vi "Tektronix_AWG Parse Binary AWG File.vi"() -> ()   [LabVIEW 2010]
doc: "Reads an array of data from a byte stream binary file. By default, the VI is configured to read 8-byte (data type DBL) Little Endian Data. To modify the way sample data is read from the file, change the Byte Order and the value of the Byte Size (normal sizes are 1, 2, 4, or 8). If you change the byte size, also change the representation of the Data Type constant (default is DBL) to coincide with the byte size (1 = I8, 2 = I16, 4 = I32, 8 = DBL). Use the Write Binary File VI in this LLB to create the file.\n\nThis example was built using LabVIEW 8.0"
panel:
  in  "Include Data Bytes as 2nd Column":bool
  out "error out":errorcluster
  in  "read file path (.awg)":path=path "c:/data/sequences/Setup1.awg"
  in  "Save As Text File?\n(will prompt for path)":bool
  out "Data":string[](array[string])
  out "Size in bytes":u32[](array[numeric])
  out "Name":string[](array[string])
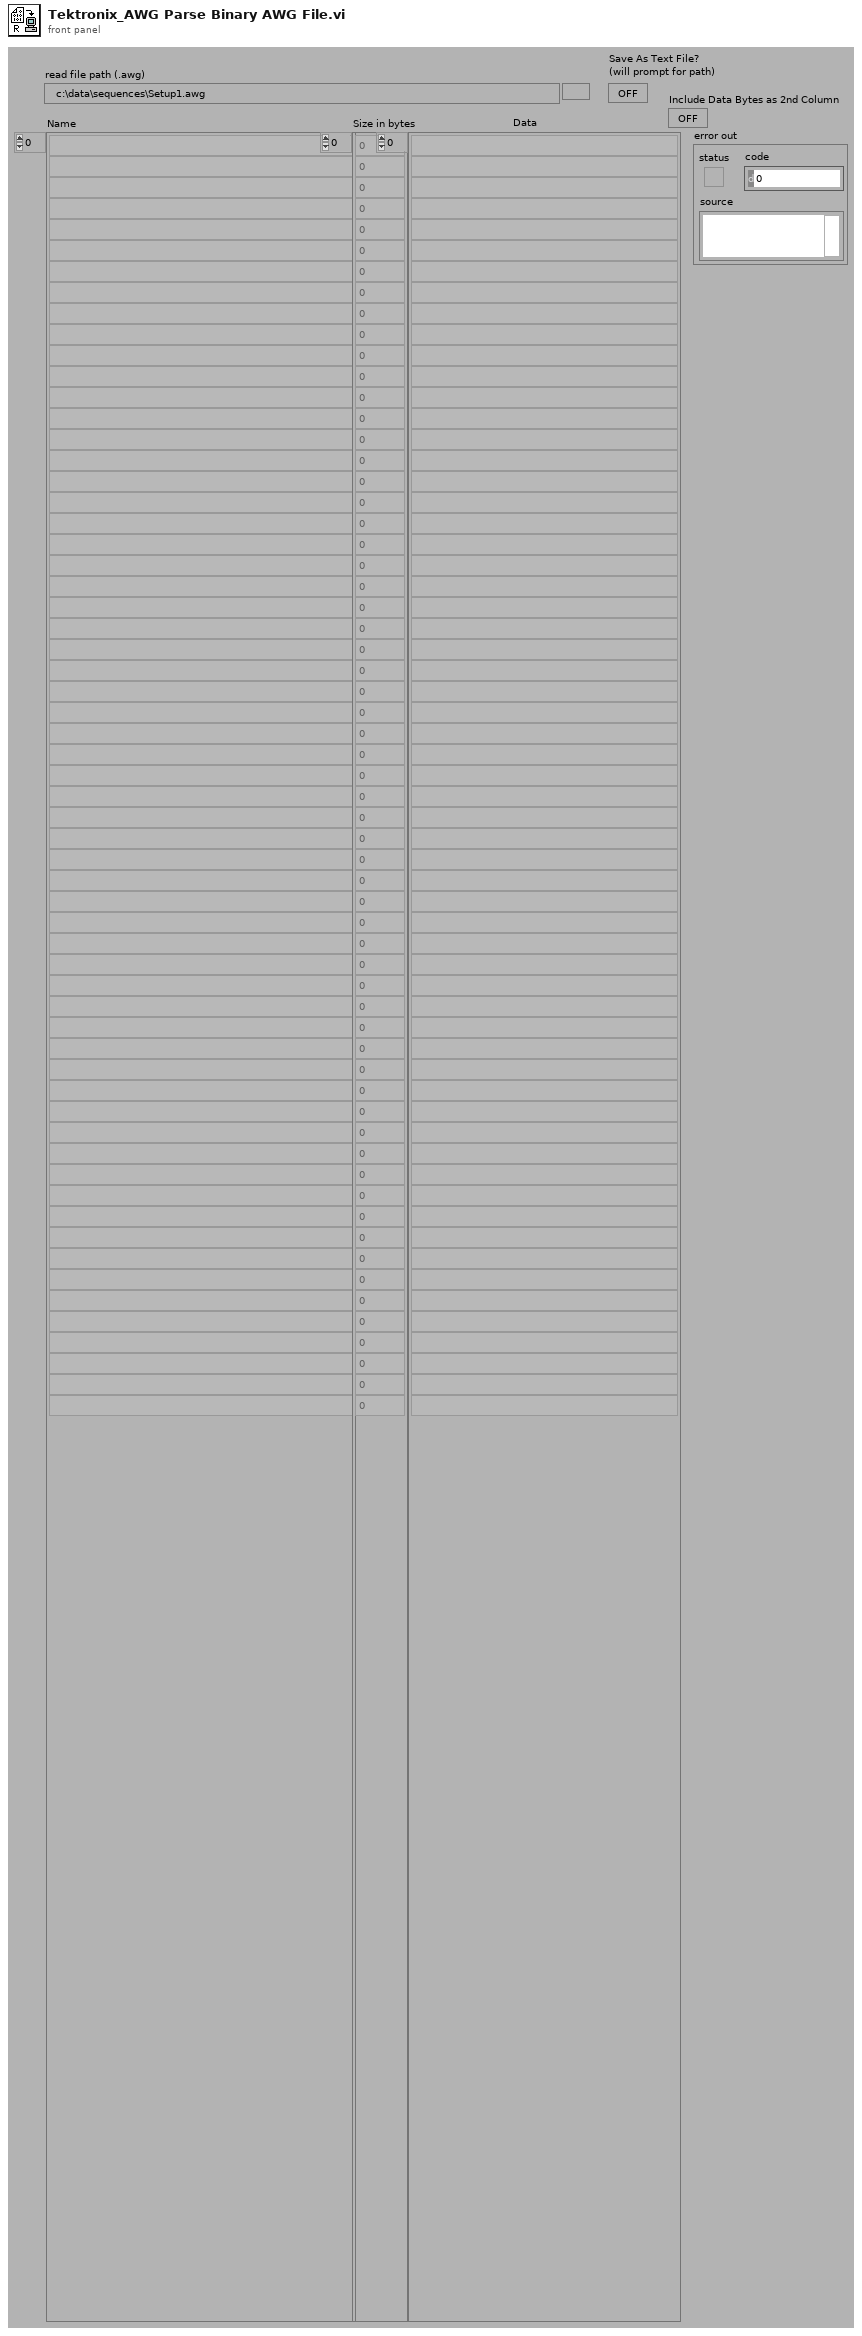
[diagram p1: front panel]
types:
  T1 = enum16{"open", "replace", "create", "open or create", "replace or create", "replace or create with confirmation"}
  T2 = enum16{"deny read/write", "deny write-only", "deny none"}
  T3 = enum16{"big-endian, network order", "native, host order", "little-endian"}
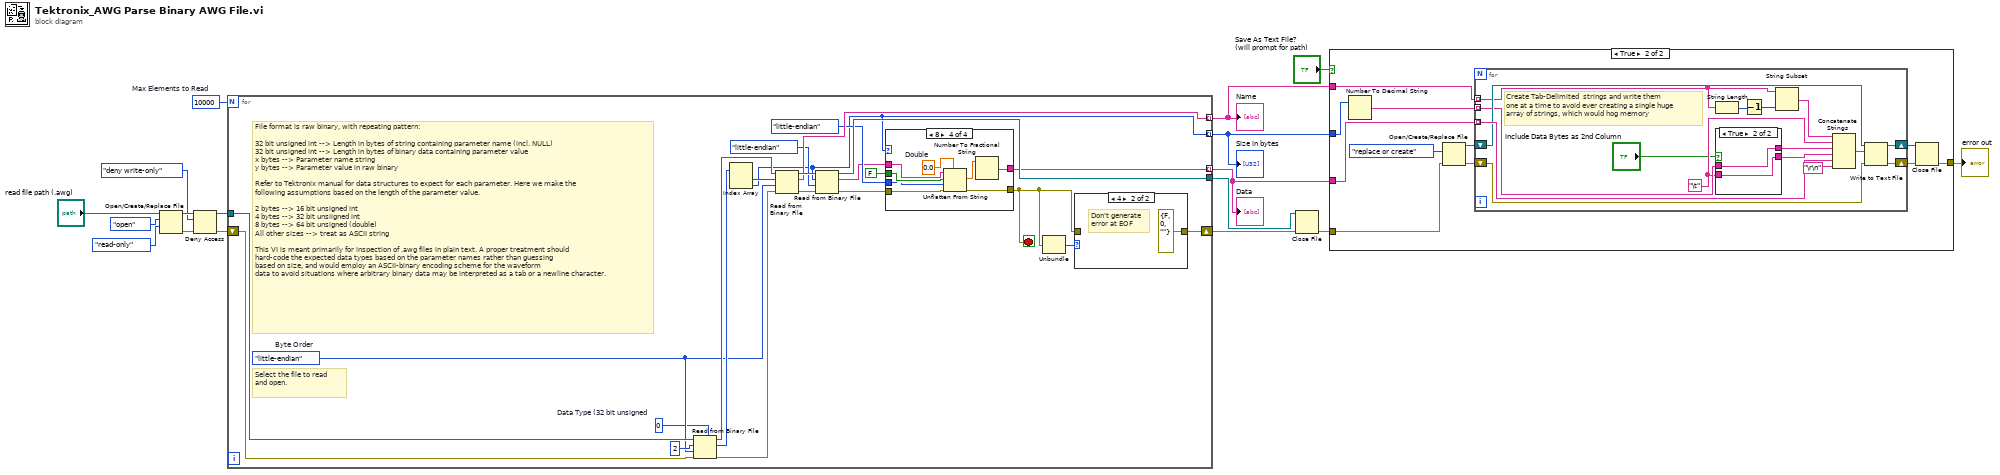
[diagram p0: block diagram]
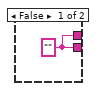
[diagram p3: hidden frame]
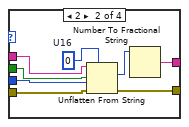
[diagram p6: hidden frame]
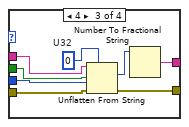
[diagram p7: hidden frame]
diagram:
  w7 = 10000  # Max Elements to Read
  n1 = Open/Create/Replace File(file path (use dialog)="read file path (.awg)", operation (0:open)=T1."open", access (0:read/write)=enum16{"read/write", "read-only", "write-only"}."read-only") -> (refnum out=w15:refnum<file>, error out=w16:errorcluster)  [unwired: 3 in, 1 out]
  n2 = Deny Access(4:w16, 6:T2."deny write-only" ("deny mode (0:deny read/write)"), 7:w15) -> (0:w11:errorcluster, 3:w12:refnum<file>)
  n3 = for {
    N: w7 -> [_]
    tunnel: w12 -> [w40]
    tunnel: [w32] -> w9
    tunnel: [w29] -> w6 mode=indexing
    tunnel: [w22] -> w5 mode=indexing
    tunnel: [w21] -> w4 mode=indexing
    shift-right: [w18] -> w8
    shift-left: w11 -> [w38]
    stop <- w19 stop-if-true
    w30 = T3."little-endian"  # Byte Order
    w28 = u32 0  # Data Type (32 bit unsigned
    # "File format is raw binary, with repeating pattern:\n\n32 bit unsigned int --> Length in bytes of string containing parameter name (incl. NULL)\n32 bit unsigned int --> Length in bytes of binary data containing parameter value\nx bytes --> Parameter name string\ny bytes --> Parameter value in raw binary\n\nRefer to Tektronix manual for data structures to expect for each parameter. Here we make the \nfollowing assumptions based on the length of the parameter value. \n\n2 bytes --> 16 bit unsigned int\n4 bytes --> 32 bit unsiigned int\n8 bytes --> 64 bit unsigned (double)\nAll other sizes --> treat as ASCII string\n\nThis VI is meant primarily for inspection of .awg files in plain text. A proper treatment should \nhard-code the expected data types based on the parameter names rather than guessing \nbased on size, and would employ an ASCII-binary encoding scheme for the waveform\ndata to avoid situations where arbitrary binary data may be interpreted as a tab or a newline character."
    # "Select the file to read and open."
    n4 = Read from Binary File(5:w28, 8:w38, 9:w30, 10:2 ("count (1)"), 11:w40) -> (0:w36:errorcluster, 2:w35:u32[], 3:w37:refnum<file>)  [unwired: 1 in, 1 out]
    n5 = Index Array(array=w35) -> (element #1=w31:u32, element #2=w22:u32)  [unwired: 2 in]
    n6 = Read from Binary File(8:w36, 9:w30, 10:w31, 11:w37) -> (0:w34:errorcluster, 2:w29:string, 3:w33:refnum<file>)  [unwired: 2 in, 1 out]
    n7 = Read from Binary File(8:w34, 9:T3."little-endian" ("byte order (0:big-endian, network order)"), 10:w22, 11:w33) -> (0:w23:errorcluster, 2:w24:string, 3:w32:refnum<file>)  [unwired: 2 in, 1 out]
    n8 = case shown="8" w22 {
      tunnel: FALSE ("data includes array or string size? (T)") -> [_ w52 w60 w68]
      tunnel: T3."little-endian" ("byte order (0:big-endian, network order)") -> [_ w51 w59 w67]
      tunnel: w24 -> [w43 w50 w58 w66]
      tunnel: w23 -> [w44 w49 w57 w65]
      tunnel: [w44 w48 w56 w64] -> w19
      tunnel: [w43 w45 w53 w61] -> w21
      frame 0, Default {
      }
      frame 2 {
        w47 = u16 0  # U16
        n9 = Unflatten From String(type=w47, binary string=w50, data includes array or string size? (T)=w52, byte order (0:big-endian, network order)=w51, error in (no error)=w49) -> (value=w46:u16, error out=w48:errorcluster)  [unwired: 1 out]
        n10 = Number To Fractional String(number=w46) -> (F-format string=w45:string)  [unwired: 3 in]
      }
      frame 4 {
        w55 = u32 0  # U32
        n11 = Unflatten From String(type=w55, binary string=w58, data includes array or string size? (T)=w60, byte order (0:big-endian, network order)=w59, error in (no error)=w57) -> (value=w54:u32, error out=w56:errorcluster)  [unwired: 1 out]
        n12 = Number To Fractional String(number=w54) -> (F-format string=w53:string)  [unwired: 3 in]
      }
      frame 8 {
        w63 = 0.0  # Double
        n13 = Unflatten From String(type=w63, binary string=w66, data includes array or string size? (T)=w68, byte order (0:big-endian, network order)=w67, error in (no error)=w65) -> (value=w62:dbl, error out=w64:errorcluster)  [unwired: 1 out]
        n14 = Number To Fractional String(number=w62) -> (F-format string=w61:string)  [unwired: 3 in]
      }
    }
    n15 = Unbundle(w19) -> ("code"=w20:i32)  [unwired: 2 out]
    n16 = case shown="4" w20 {
      tunnel: w19 -> [w41 _]
      tunnel: [w41 errorcluster {"status"=FALSE, "code"=0, "source"=""} ("error out")] -> w18
      frame 0, Default {
      }
      frame 4 {
        # "Don't generate\nerror at EOF"
      }
    }
  }
  "Name" <- w6
  "Size in bytes" <- w5
  "Data" <- w4
  n17 = Close File(refnum=w9, error in=w8) -> (error out=w2:errorcluster)  [unwired: 1 out]
  n18 = case shown="True" "Save As Text File?\n(will prompt for path)" {
    tunnel: w6 -> [_ w80]
    tunnel: w5 -> [_ w79]
    tunnel: w4 -> [_ w77]
    tunnel: w2 -> [w69 w76]
    tunnel: [w69 w72] -> w1
    frame False {
    }
    frame True {
      n19 = Number To Decimal String(number=w79) -> (decimal integer string=w78:string[])  [unwired: 1 in]
      n20 = Open/Create/Replace File(error in=w76, operation (0:open)=T1."replace or create") -> (refnum out=w74:refnum<file>, error out=w75:errorcluster)  [unwired: 4 in, 1 out]
      n21 = for {
        tunnel: w80 -> [w89] mode=indexing
        tunnel: w78 -> [w85] mode=indexing
        tunnel: w77 -> [w96] mode=indexing
        shift-right: [w91] -> w73
        shift-left: w74 -> [w94]
        shift-right: [w90] -> w71
        shift-left: w75 -> [w93]
        w83 = "\t"
        # "Create Tab-Delimited  strings and write them\none at a time to avoid ever creating a single huge \narray of strings, which would hog memory"
        n22 = String Length(string=w89) -> (length=w88:i32)
        n23 = case shown="True" "Include Data Bytes as 2nd Column" {
          tunnel: w85 -> [_ w99]
          tunnel: [w97 w99] -> w84
          tunnel: w83 -> [_ w98]
          tunnel: [w97 w98] -> w82
          frame False {
            w97 = "" ("Data Type (32 bit unsigned")
          }
          frame True {
          }
        }
        n24 = Decrement(x=w88) -> (x-1=w87:i32)
        n25 = String Subset(string=w89, length (rest)=w87) -> (substring=w86:string)  [unwired: 1 in]
        n26 = Concatenate Strings(w86, w83, w84, w82, w96, "\r\n") -> (w92:string)
        n27 = Write to Text File(file (use dialog)=w94, text=w92, error in=w93) -> (refnum out=w91:refnum<file>, error out=w90:errorcluster)  [unwired: 1 in, 1 out]
      }
      n28 = Close File(refnum=w73, error in=w71) -> (error out=w72:errorcluster)  [unwired: 1 out]
    }
  }
  "error out" <- w1
